vi "RotationMatrixBetweenPlanes.vi"(8 "error in":errorcluster, 9 "Plane 2 Coeffcients":T1, 11 "Plane 1 Coeffcients":T1) -> (0 "error out":errorcluster, 3 "Rotation Matrix":T2)   [LabVIEW 2020, in "pointset_utils.lvlib" / "Align Point Set to Plane.lvlib"]
uses:
  Align Point Set to Plane.lvlib
  PlaneCoeffecients.ctl
  <vilib>/Analysis/Matrix/Datatypes/RealMatrix.ctl
  <vilib>/Analysis/baseanly.llb/Real Dot Product.vi
  <vilib>/Analysis/7linalg.llb/Real Matrix Power.vi
  <vilib>/Analysis/_algsub.llb/Real Matrix Norm.vi
  <vilib>/Analysis/7linalg.llb/Create Special Real Matrix.vi
  <vilib>/Analysis/Matrix/NI_Matrix.lvlib
  <vilib>/Analysis/NI_AALPro.lvlib
  <vilib>/Analysis/NI_AALBase.lvlib
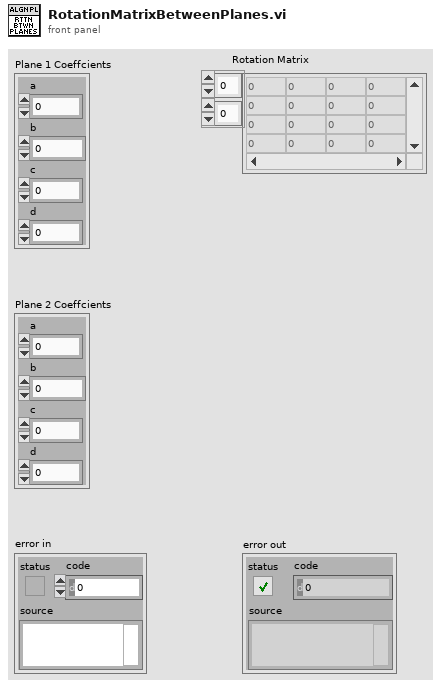
[diagram p1: front panel]
types:
  T1 = typedef "pointset_utils.lvlib/Align Point Set to Plane.lvlib/PlaneCoeffecients.ctl" = cluster{"a":dbl, "b":dbl, "c":dbl, "d":dbl}
  T2 = typedef "NI_Matrix.lvlib/RealMatrix.ctl" = dbl[][]
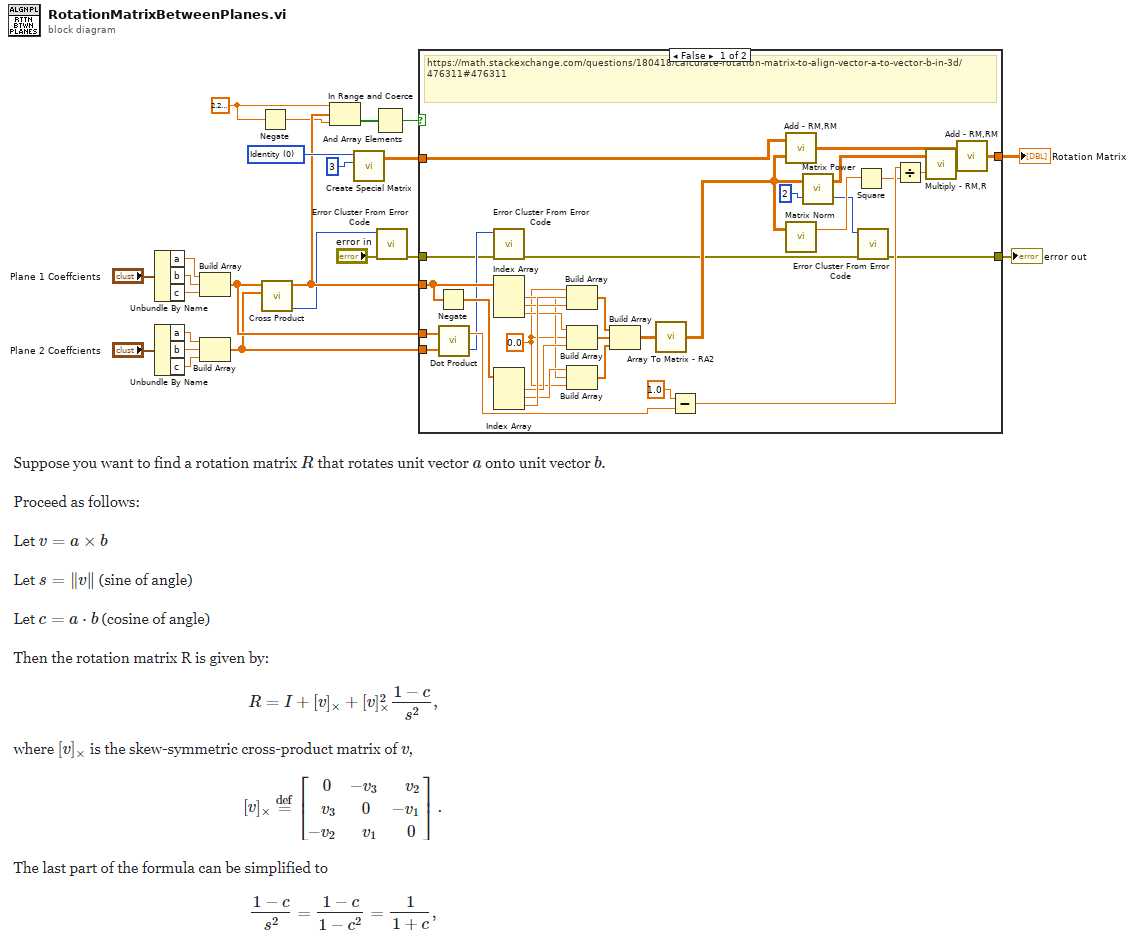
[diagram p0: block diagram]
diagram:
  w13 = 2.220446049250313e-16
  w23 = 0 items=["Identity", "Diagonal", "Toeplitz", "Vandermonde", "Companion", "Hankel", "Hadamard", "Wilkinson", "Hilbert", "Inverse Hilbert", "Rosser", "Pascal"] ("matrix type")
  n1 = Unbundle By Name("Plane 1 Coeffcients") -> ("a"=w20:dbl, "b"=w19:dbl, "c"=w18:dbl)
  n2 = Unbundle By Name("Plane 2 Coeffcients") -> ("a"=w8:dbl, "b"=w7:dbl, "c"=w6:dbl)
  n3 = Build Array(w20, w19, w18) -> (w17:dbl[])
  n4 = Build Array(w8, w7, w6) -> (w5:dbl[])
  n5 = Negate(x=w13) -> (-x=w12:dbl)
  n6 = call <vilib>:"Cross Product.vi"("B Vector"=w5, "A Vector"=w17) -> ("error"=w4:i32, "Cross Product"=w14:dbl[])  [unwired: 8 in]
  n7 = In Range and Coerce(upper limit=w13, x=w14, lower limit=w12) -> (In Range?=w11:bool[])  [unwired: 1 out]
  n8 = call-poly <vilib>:"Create Special Matrix.vi"("matrix type"=w23, "matrix size"=3) -> ("Special Matrix"=w21:T2)  [unwired: 3 in, 1 out]
  n9 = And Array Elements(Boolean array=w11) -> (logical AND=w10:bool)
  n10 = call <vilib>:"Error Cluster From Error Code.vi"("error in (no error)"="error in", "error code (0)"=w4) -> ("error out"=w3:errorcluster)  [unwired: 7 in]
  n11 = case shown="False" w10 {
    tunnel: w21 -> [w55 w58]
    tunnel: w17 -> [w44 _]
    tunnel: w5 -> [w43 _]
    tunnel: [w30 w58] -> w15
    tunnel: w14 -> [w29 _]
    tunnel: w3 -> [w26 w57]
    tunnel: [w24 w57] -> w1
    frame False {
      w35 = 0.0 ("element")
      # "https://math.stackexchange.com/questions/180418/calculate-rotation-matrix-to-align-vector-a-to-vector-b-in-3d/476311#476311"
      n12 = Negate(x=w29) -> (-x=w42:dbl[])
      n13 = call-poly <vilib>:"Dot Product.vi"("Y Vector"=w43, "X Vector"=w44) -> ("error"=w28:i32, "X * Y"=w53:dbl)
      n14 = call <vilib>:"Error Cluster From Error Code.vi"("error in (no error)"=w26, "error code (0)"=w28) -> ("error out"=w25:errorcluster)  [unwired: 7 in]
      n15 = Index Array(array=w29) -> (element #1=w36:dbl, element #2=w40:dbl, element #3=w39:dbl)  [unwired: 3 in]
      n16 = Index Array(array=w42) -> (element #1=w38:dbl, element #2=w37:dbl, element #3=w41:dbl)  [unwired: 3 in]
      n17 = Build Array(w35, w41, w40) -> (w32:dbl[])
      n18 = Build Array(w39, w35, w38) -> (w33:dbl[])
      n19 = Build Array(w37, w36, w35) -> (w34:dbl[])
      n20 = Build Array(w32, w33, w34) -> (w31:dbl[][])
      n21 = call <vilib>:"Array To Matrix - RA2.vi"("Real 2D Array"=w31) -> ("Real Matrix"=w50:T2)
      n22 = Subtract(x=1.0, y=w53) -> (x-y=w52:dbl)
      n23 = call <vilib>:"Add - RM,RM.vi"("Real Matrix B"=w50, "Real Matrix A"=w55) -> ("A + B"=w49:T2)
      n24 = call-poly <vilib>:"Matrix Norm.vi"("Input Matrix"=w50) -> ("norm"=w47:dbl)  [unwired: 1 in, 1 out]
      n25 = call-poly <vilib>:"Matrix Power.vi"("n"=2, "Input Matrix"=w50) -> ("error"=w27:i32, "Matrix Power"=w51:T2)
      n26 = Square(x=w47) -> (x^2=w46:dbl)
      n27 = call <vilib>:"Error Cluster From Error Code.vi"("error in (no error)"=w25, "error code (0)"=w27) -> ("error out"=w24:errorcluster)  [unwired: 7 in]
      n28 = Divide(x=w52, y=w46) -> (x/y=w45:dbl)
      n29 = call <vilib>:"Multiply - RM,R.vi"("Real Scalar c"=w45, "Real Matrix A"=w51) -> ("A * c"=w48:T2)
      n30 = call <vilib>:"Add - RM,RM.vi"("Real Matrix B"=w48, "Real Matrix A"=w49) -> ("A + B"=w30:T2)
    }
    frame True {
      # "Planes Already Aligned"
    }
  }
  "Rotation Matrix" <- w15
  "error out" <- w1
